vi "YawOverflows.vi"(1 "Yaw (radians)":dbl) -> (0 "Yaw (with overflows)":dbl)   [LabVIEW 2015]
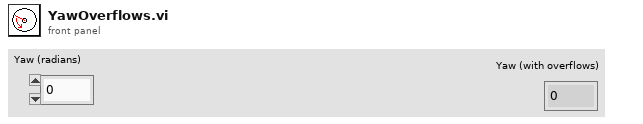
[diagram p1: front panel]
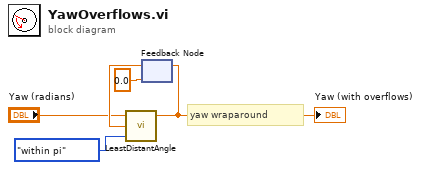
[diagram p0: block diagram]
diagram:
  # "yaw wraparound"
  n1 = feedback #1(0.0) -> (w3:dbl)
  n2 = call "LeastDistantAngle.vi"("Enum"=enum16{"within pi", "within pi/2"}."within pi", "Current angle"=w3, "target angle (between pi and -pi)"="Yaw (radians)") -> ("output angle"=w1:dbl)  [unwired: 2 out]
  "Yaw (with overflows)" <- w1
  n3 = feedback-in #1(w1) -> ()
